vi "Transmit-state.vi"(8 "error in (no error)":errorcluster, 9 "X2":dbl, 10 "X1":dbl, 11 "XNET Session":refnum<k21>="Plant2_state") -> (0 "error out":errorcluster)   [LabVIEW 2016]
uses:
  Tolerance.ctl
  <vilib>/xnet/xnet.llb/XNET Write (Signal Single-point).vi
  <vilib>/Analysis/_algsub.llb/Real Vector Norm.vi
  <vilib>/Analysis/NI_AALPro.lvlib
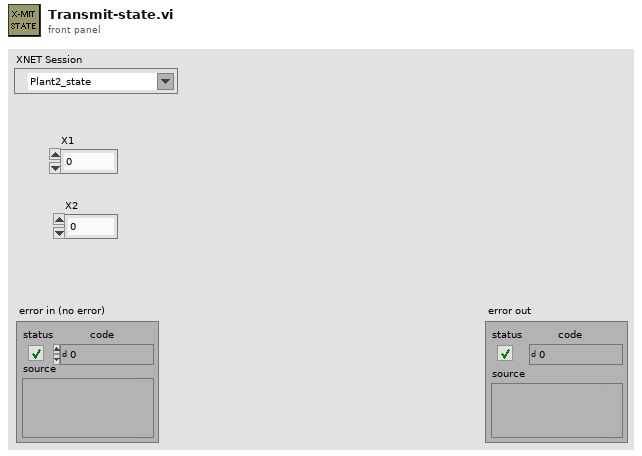
[diagram p1: front panel]
types:
  T1 = typedef "Tolerance.ctl" = dbl
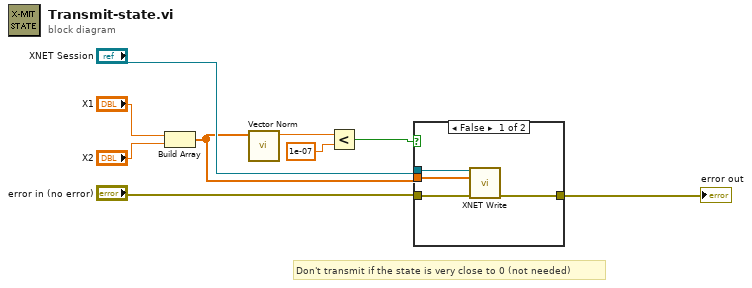
[diagram p0: block diagram]
diagram:
  # "Don't transmit if the state is very close to 0 (not needed)"
  n1 = Build Array("X1", "X2") -> (w4:dbl[])
  n2 = call-poly <vilib>:"Vector Norm.vi"("Input Vector"=w4) -> ("norm"=w3:dbl)  [unwired: 9 in, 1 out]
  n3 = Less?(x=w3, y=T1 1e-07 ("Tolerance")) -> (x < y?=w1:bool)
  n4 = case shown="False" w1 {
    tunnel: "XNET Session" -> [w13 _]
    tunnel: "error in (no error)" -> [w12 w14]
    tunnel: [w11 w14] -> w5
    tunnel: w4 -> [w10 _]
    frame False {
      n5 = call-poly <vilib>:"XNET Write.vi"("session in"=w13, "data"=w10, "error in (no error)"=w12) -> ("error out"=w11:errorcluster)  [unwired: 11 in, 1 out]
    }
    frame True {
    }
  }
  "error out" <- w5
